vi "GRAPH TO ARRAY ATTRIBUTES.vi"(11 "input cluster":T1) -> (3 "Array":u32[](array[numeric]))   [LabVIEW 2014]
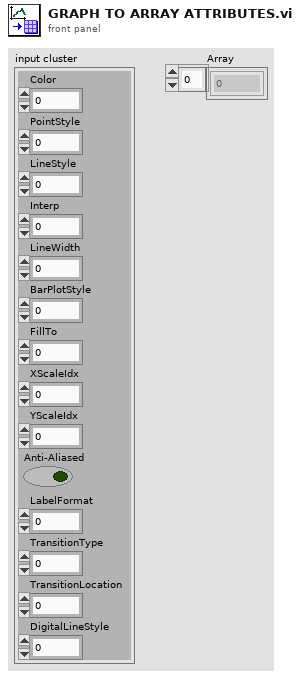
[diagram p1: front panel]
types:
  T1 = cluster{"Color":u32, "PointStyle":u8, "LineStyle":u8, "Interp":u8, "LineWidth":u8, "BarPlotStyle":u8, "FillTo":i16, "XScaleIdx":u32, "YScaleIdx":u32, "Anti-Aliased":bool, "LabelFormat":u8, "TransitionType":u8, "TransitionLocation":u8, "DigitalLineStyle":u8}
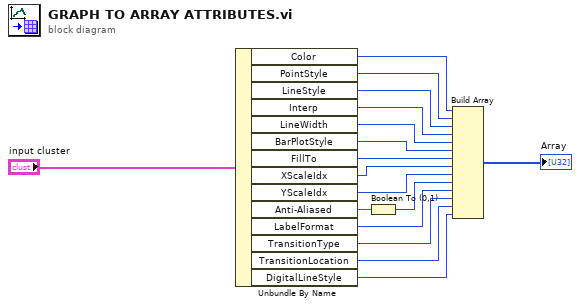
[diagram p0: block diagram]
diagram:
  n1 = Unbundle By Name("input cluster") -> ("Color"=w3:u32, "PointStyle"=w4:u8, "LineStyle"=w5:u8, "Interp"=w6:u8, "LineWidth"=w7:u8, "BarPlotStyle"=w8:u8, "FillTo"=w9:i16, "XScaleIdx"=w10:u32, "YScaleIdx"=w11:u32, "Anti-Aliased"=w2:bool, "LabelFormat"=w13:u8, "TransitionType"=w14:u8, "TransitionLocation"=w15:u8, "DigitalLineStyle"=w16:u8)
  n2 = Boolean To (0,1)(Boolean=w2) -> (0, 1=w12:i16)
  n3 = Build Array(w3, w4, w5, w6, w7, w8, w9, w10, w11, w12, w13, w14, w15, w16) -> (→"Array":u32[])
